vi "NXT_ Init Sensor Data.vi"() -> (0 "_sensorData":T1)   [LabVIEW 2012, in "Tugboat.lvrbt"]
uses:
  Tugboat.lvrbt
  sensorData_t.ctl
  irData_t.ctl
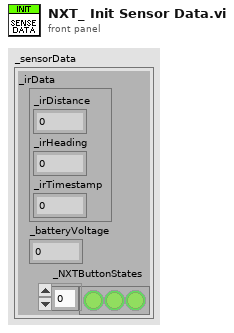
[diagram p1: front panel]
types:
  T1 = typedef "sensorData_t.ctl" = cluster{"_irData":T2, "_batteryVoltage":i32, "_NXTButtonStates":bool[]}
  T2 = typedef "irData_t.ctl" = cluster{"_irDistance":i32, "_irHeading":i32, "_irTimestamp":u32}
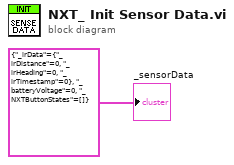
[diagram p0: block diagram]
diagram:
  "_sensorData" <- T1 {"_irData"={"_irDistance"=0, "_irHeading"=0, "_irTimestamp"=0}, "_batteryVoltage"=0, "_NXTButtonStates"=[]} ("_sensorData")
